vi "GetColumns.vi"(8 "error in (no error)":errorcluster, 11 "XML":string) -> (0 "error out":errorcluster, 3 "#Columns":i32)   [LabVIEW 2014]
uses:
  XML.lvlib
  <resource>/objmgr/DOMUserDefRef.rc
panel:
  # "Input"
  # "Output"
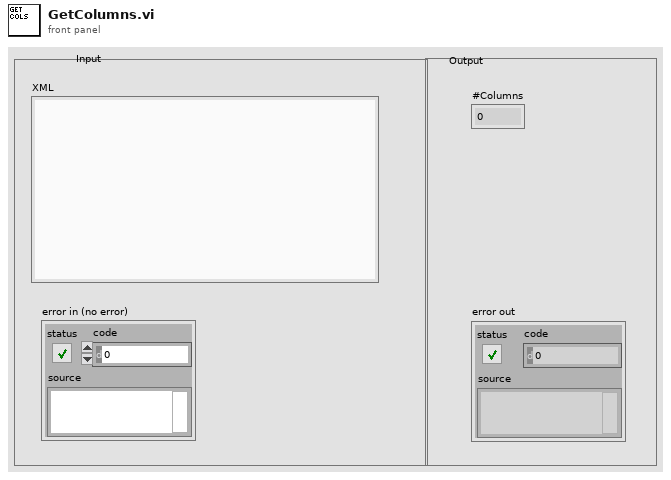
[diagram p1: front panel]
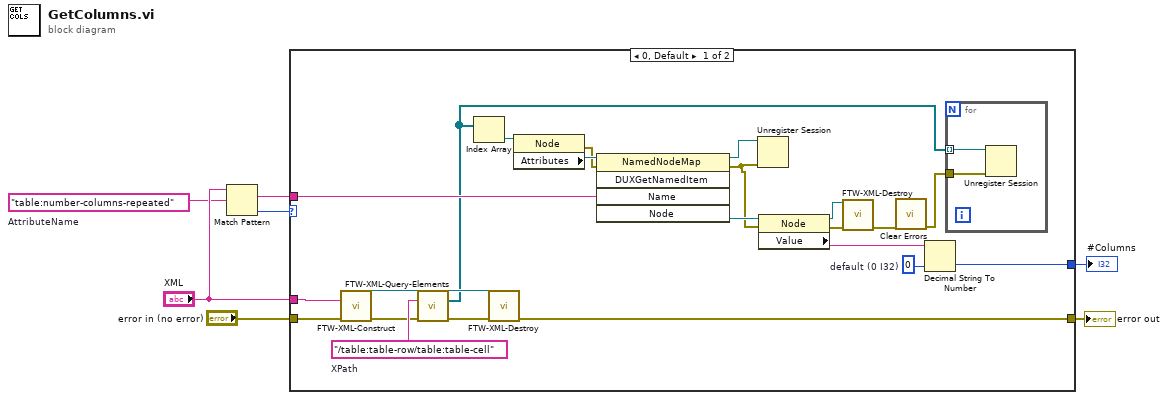
[diagram p0: block diagram]
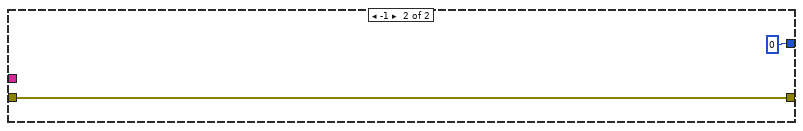
[diagram p2: hidden frame]
diagram:
  w4 = "table:number-columns-repeated"  # AttributeName
  n1 = Match Pattern(string="XML", regular expression=w4) -> (match substring=w3:string, offset past match=w2:i32)  [unwired: 1 in, 2 out]
  n2 = case shown="0, Default" w2 {
    tunnel: [w28 0] -> w7
    tunnel: "error in (no error)" -> [w22 w33]
    tunnel: "XML" -> [w19 _]
    tunnel: w3 -> [w18 _]
    tunnel: [w17 w33] -> w1
    frame 0, Default {
      w16 = 0  # default (0 I32)
      w30 = "/table:table-row/table:table-cell"  # XPath
      n3 = call "FTW-XML-Construct.vi"("XML String"=w19, "error in"=w22) -> ("XML Document"=w20:refnum<k20>, "error out"=w21:errorcluster)  [unwired: 12 in]
      n4 = call "FTW-XML-Query-Elements.vi"("XML Node"=w20, "XPath Query"=w30, "error in"=w21) -> ("XML Node out"=w23:refnum<k20>, "Matching Nodes"=w13:refnum<k20>[], "error out"=w24:errorcluster)  [unwired: 9 in, 1 out]
      n5 = Index Array(array=w13) -> (element=w29:refnum<k20>)  [unwired: 1 in]
      n6 = call "FTW-XML-Destroy.vi"("XML Node"=w23, "error in"=w24) -> ("error out"=w17:errorcluster)  [unwired: 13 in]
      n7 = property class="Node"(reference=w29) -> (error out=w15:errorcluster, "Attributes"=w25:refnum<k20>)  [unwired: 1 in, 1 out]
      n8 = invoke class="NamedNodeMap" method="DUXGetNamedItem"(reference=w25, error in=w15, "Name"=w18) -> (reference out=w8:refnum<k20>, error out=w9:errorcluster, "Node"=w27:refnum<k20>)  [unwired: 2 in, 2 out]
      n9 = Unregister Session(8:w9, 11:w8) -> ()  [unwired: 1 out]
      n10 = property class="Node"(reference=w27, error in=w9) -> (reference out=w12:refnum<k20>, error out=w11:errorcluster, "Value"=w26:string)
      n11 = call "FTW-XML-Destroy.vi"("XML Node"=w12, "error in"=w11) -> ("error out"=w10:errorcluster)  [unwired: 13 in]
      n12 = call <vilib>:"Clear Errors.vi"("error in (no error)"=w10) -> ("error out"=w14:errorcluster)  [unwired: 5 in, 1 out]
      n13 = Decimal String To Number(string=w26, default (0L)=w16) -> (number=w28:i32)  [unwired: 1 in, 1 out]
      n14 = for {
        tunnel: w14 -> [w32]
        tunnel: w13 -> [w31] mode=indexing
        n15 = Unregister Session(8:w32, 11:w31) -> ()  [unwired: 1 out]
      }
    }
    frame -1 {
    }
  }
  "#Columns" <- w7
  "error out" <- w1
